vi "Distance Calcuator.vi"() -> ()   [LabVIEW 2015]
panel:
  out "Horizontal Fill Slide 2":dbl(slide) scale=0.0..70.0
  out "x/y":dbl
  in  "x":dbl format="%#_13g"
  out "Circles (Shape Detection 1)":T1(array[cluster]) {"Position"."Y" format="%.2f"; "Position"."X" format="%.2f"}
  out "fps":dbl(knob) scale=0.0..30.0
  out "Frame Rate":dbl
  in  "Stop (F)":bool
  out "Image Out":T2(plugin-control)
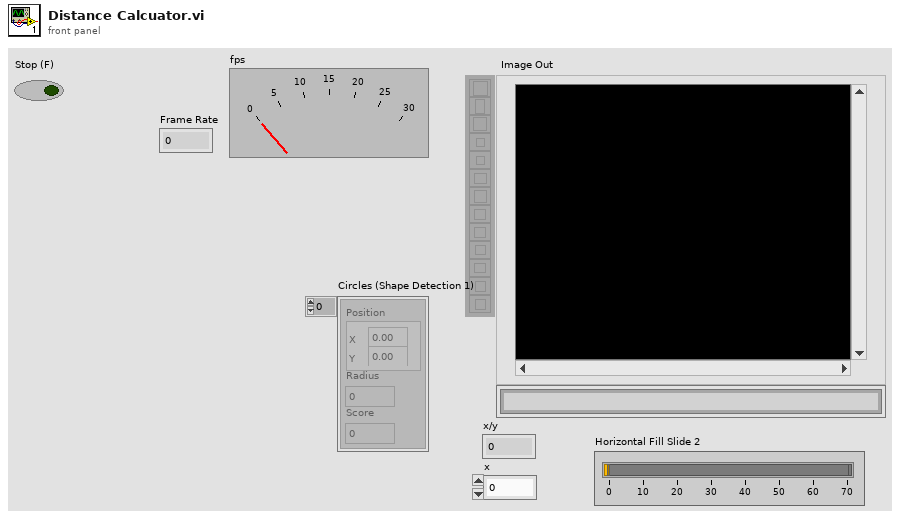
[diagram p1: front panel]
types:
  T1 = cluster{"Position":cluster{"X":sgl, "Y":sgl}, "Radius":dbl, "Score":dbl}[]
  T2 = typedef "IMAQ Image.ctl" = refnum<image>
  T3 = cluster{"Circles (Shape Detection 1)[0]":cluster{"Position":cluster{"X":sgl, "Y":sgl}, "Radius":dbl, "Score":dbl}, "Circles (Shape Detection 1)[1]":cluster{"Position":cluster{"X":sgl, "Y":sgl}, "Radius":dbl, "Score":dbl}, "Circles (Shape Detection 1)[2]":cluster{"Position":cluster{"X":sgl, "Y":sgl}, "Radius":dbl, "Score":dbl}, "Circles (Shape Detection 1)[3]":cluster{"Position":cluster{"X":sgl, "Y":sgl}, "Radius":dbl, "Score":dbl}, "Circles (Shape Detection 1)[4]":cluster{"Position":cluster{"X":sgl, "Y":sgl}, "Radius":dbl, "Score":dbl}, "Circles (Shape Detection 1)[5]":cluster{"Position":cluster{"X":sgl, "Y":sgl}, "Radius":dbl, "Score":dbl}, "Circles (Shape Detection 1)[6]":cluster{"Position":cluster{"X":sgl, "Y":sgl}, "Radius":dbl, "Score":dbl}, "Circles (Shape Detection 1)[7]":cluster{"Position":cluster{"X":sgl, "Y":sgl}, "Radius":dbl, "Score":dbl}, "Circles (Shape Detection 1)[8]":cluster{"Position":cluster{"X":sgl, "Y":sgl}, "Radius":dbl, "Score":dbl}}
  T4 = cluster{"Position":cluster{"X":sgl, "Y":sgl}, "Radius":dbl, "Score":dbl}
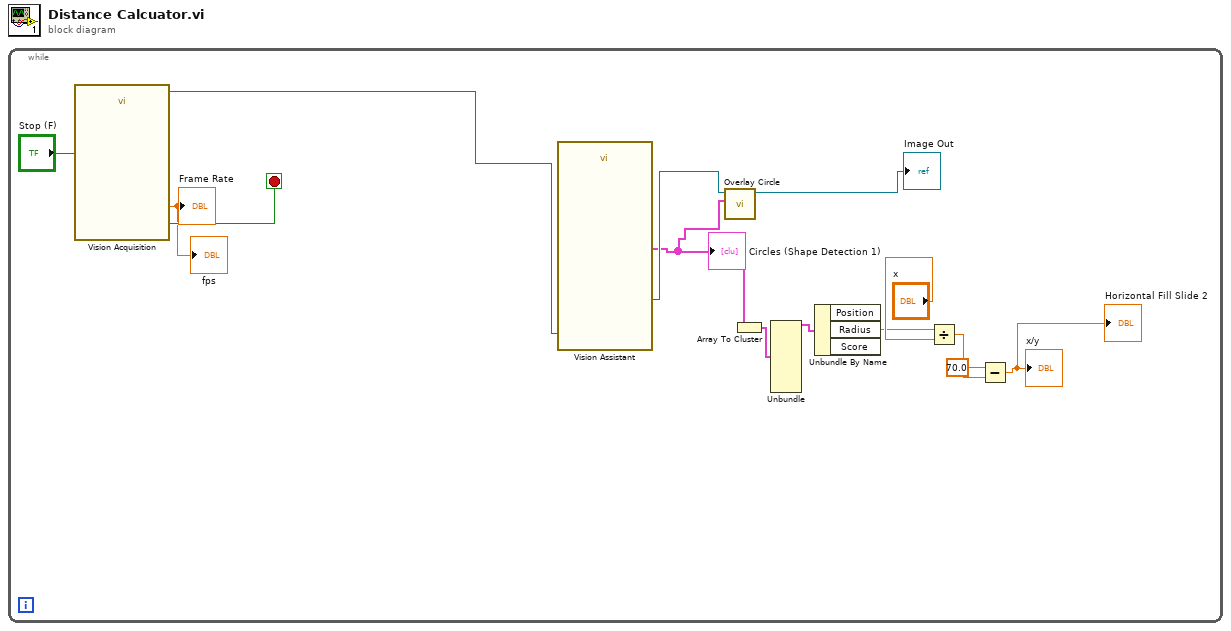
[diagram p0: block diagram]
diagram:
  n1 = while {
    stop <- w13 stop-if-true
    n2 = call "Vision Acquisition"("Stop (F)"="Stop (F)") -> ("Image Out"=w11:T2, "Frame Rate"=→"Frame Rate" →"fps":dbl, "Stopped"=w13:bool)  [unwired: 22 in, 2 out]
    n3 = call "Vision Assistant"("Image In"=w11) -> ("Image Out"=w10:T2, "Circles (Shape Detection 1)"=w8:T1)  [unwired: 22 in, 3 out]
    "Circles (Shape Detection 1)" <- w8
    n4 = call "Overlay Circle.vi"("Circles (Shape Detection 1) in"=w8, "Refnum in"=w10) -> ("Refnum out"=→"Image Out":T2)  [unwired: 7 in, 2 out]
    n5 = Array To Cluster(array=w8) -> (cluster=w7:T3)
    n6 = Unbundle(w7) -> ("Circles (Shape Detection 1)[0]"=w6:T4)  [unwired: 8 out]
    n7 = Unbundle By Name(w6) -> ("Radius"=w4:dbl)  [unwired: 2 out]
    n8 = Divide(x=w4, y="x") -> (x/y=w3:dbl)
    n9 = Subtract(x=70.0, y=w3) -> (x-y=→"x/y" →"Horizontal Fill Slide 2":dbl)
  }
